vi "Delete Buffer.vi"(11 "BufferLastReadings DBL in":refnum<class "BufferLastReadings DBL.lvclass">) -> (3 "BufferLastReadings DBL out":refnum<class "BufferLastReadings DBL.lvclass">)   [LabVIEW 2023, in "BufferLastReadings DBL.lvclass"]
uses:
  BufferLastReadings DBL.lvclass
  BufferLastReadings DBL.lvclass/BufferLastReadings DBL.ctl
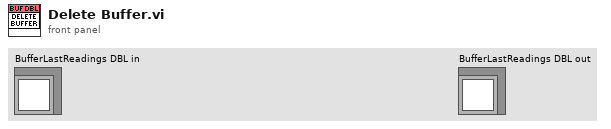
[diagram p1: front panel]
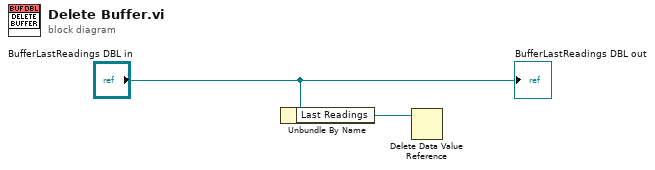
[diagram p0: block diagram]
diagram:
  n1 = Unbundle By Name("BufferLastReadings DBL in") -> ("Last Readings"=w1:refnum<data-value>)
  n2 = Delete Data Value Reference(data value reference=w1) -> ()  [unwired: 1 in, 2 out]
  "BufferLastReadings DBL out" <- "BufferLastReadings DBL in"
